vi "write_all_conditions_to_ini.vi"() -> ()   [LabVIEW 2019]
uses:
  <vilib>/Utility/config.llb/NI_LVConfig.lvlib
panel:
  in  "Conditions cluster":T1
  in  "configuration file path":path
  in  "Error in":errorcluster
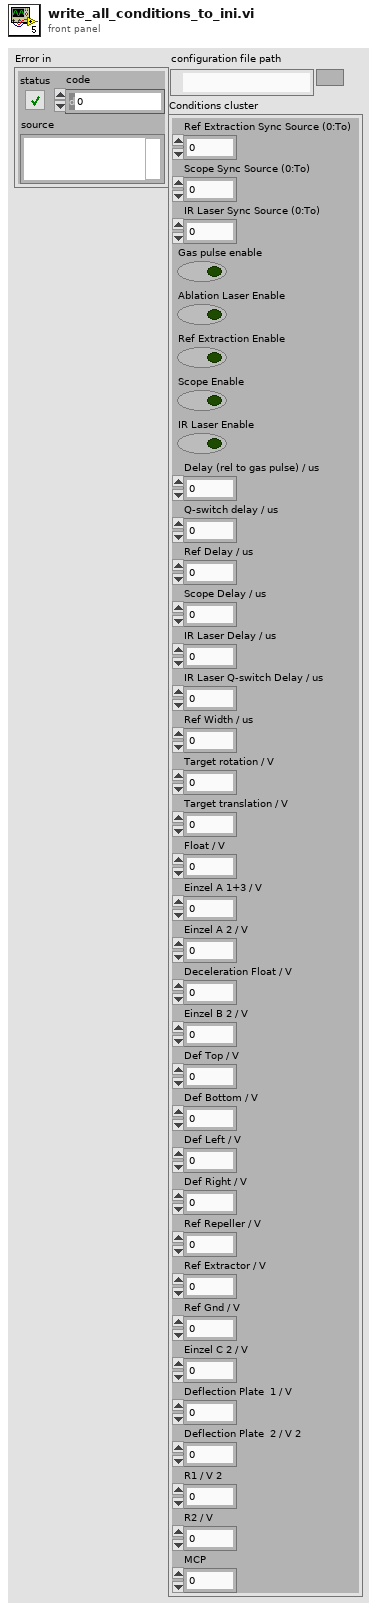
[diagram p1: front panel]
types:
  T1 = cluster{"Ref Extraction Sync Source (0:To)":i32, "Scope Sync Source (0:To)":i32, "IR Laser Sync Source (0:To)":i32, "Gas pulse enable":bool, "Ablation Laser Enable":bool, "Ref Extraction Enable":bool, "Scope Enable":bool, "IR Laser Enable":bool, "Delay (rel to gas pulse) / us":dbl, "Q-switch delay / us":dbl, "Ref Delay / us":dbl, "Scope Delay / us":dbl, "IR Laser Delay / us":dbl, "IR Laser Q-switch Delay / us":dbl, "Ref Width / us":dbl, "Target rotation / V":dbl, "Target translation / V":dbl, "Float / V":dbl, "Einzel A 1+3 / V":dbl, "Einzel A 2 / V":dbl, "Deceleration Float / V":dbl, "Einzel B 2 / V":dbl, "Def Top / V":dbl, "Def Bottom / V":dbl, "Def Left / V":dbl, "Def Right / V":dbl, "Ref Repeller / V":dbl, "Ref Extractor / V ":dbl, "Ref Gnd / V ":dbl, "Einzel C 2 / V":dbl, "Deflection Plate  1 / V":dbl, "Deflection Plate  2 / V 2":dbl, "R1 / V 2":dbl, "R2 / V":dbl, "MCP":dbl}
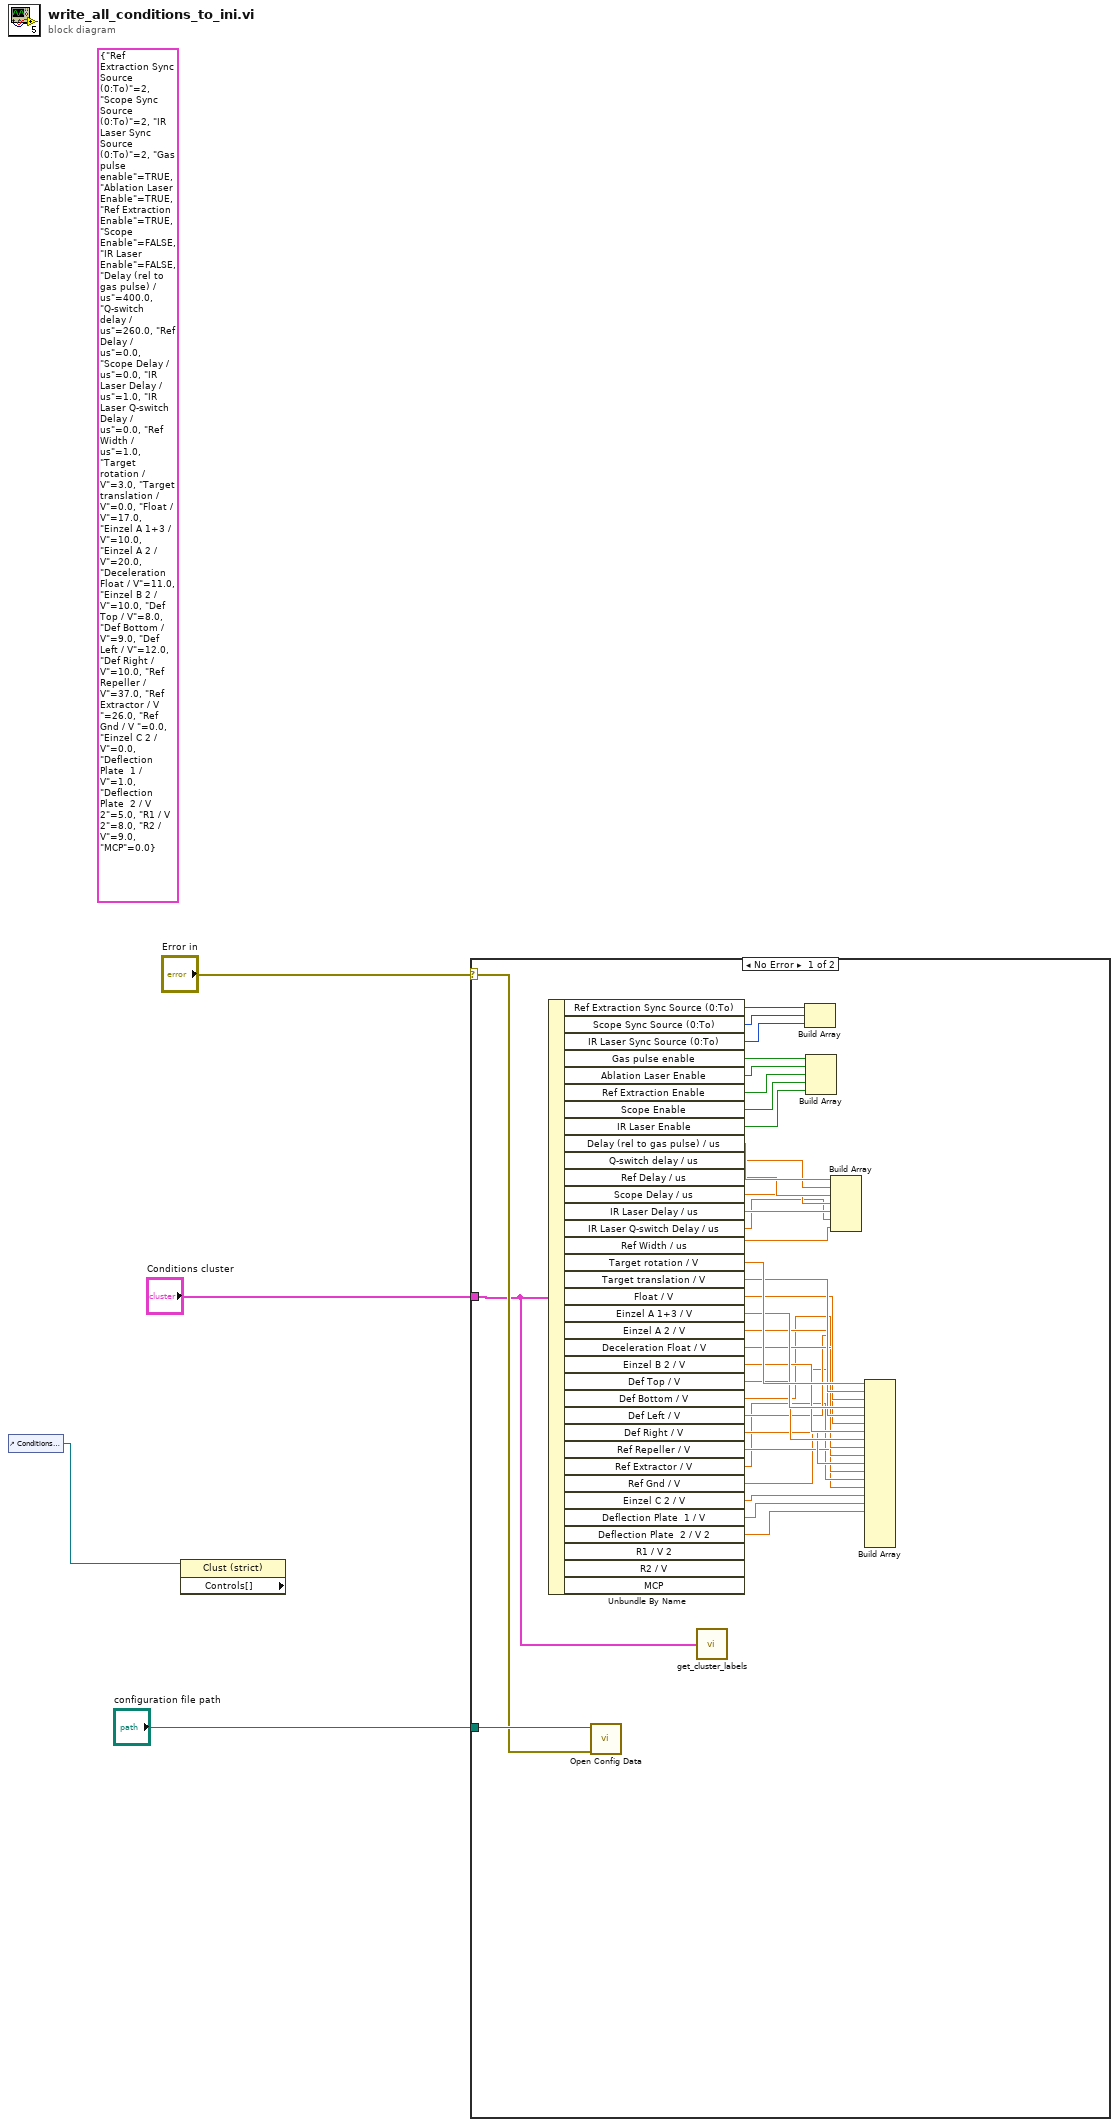
[diagram p0: block diagram]
diagram:
  (unwired) T1 {"Ref Extraction Sync Source (0:To)"=2, "Scope Sync Source (0:To)"=2, "IR Laser Sync Source (0:To)"=2, "Gas pulse enable"=TRUE, "Ablation Laser Enable"=TRUE, "Ref Extraction Enable"=TRUE, "Scope Enable"=FALSE, "IR Laser Enable"=FALSE, "Delay (rel to gas pulse) / us"=400.0, "Q-switch delay / us"=260.0, "Ref Delay / us"=0.0, "Scope Delay / us"=0.0, "IR Laser Delay / us"=1.0, "IR Laser Q-switch Delay / us"=0.0, "Ref Width / us"=1.0, "Target rotation / V"=3.0, "Target translation / V"=0.0, "Float / V"=17.0, "Einzel A 1+3 / V"=10.0, "Einzel A 2 / V"=20.0, "Deceleration Float / V"=11.0, "Einzel B 2 / V"=10.0, "Def Top / V"=8.0, "Def Bottom / V"=9.0, "Def Left / V"=12.0, "Def Right / V"=10.0, "Ref Repeller / V"=37.0, "Ref Extractor / V "=26.0, "Ref Gnd / V "=0.0, "Einzel C 2 / V"=0.0, "Deflection Plate  1 / V"=1.0, "Deflection Plate  2 / V 2"=5.0, "R1 / V 2"=8.0, "R2 / V"=9.0, "MCP"=0.0} ("input cluster")
  n1 = control-ref of="Conditions cluster"() -> (w1:refnum<vi>)
  n2 = property class="Clust (strict)" props=["Controls[]"](reference=w1) -> ()  [unwired: 1 in, 3 out]
  n3 = case shown="No Error" "Error in" {
    selector: "Error in" -> [w38 _]
    tunnel: "configuration file path" -> [w39 _]
    tunnel: "Conditions cluster" -> [w37 _]
    frame No Error {
      n4 = Unbundle By Name(w37) -> ("Ref Extraction Sync Source (0:To)"=w36:i32, "Scope Sync Source (0:To)"=w35:i32, "IR Laser Sync Source (0:To)"=w34:i32, "Gas pulse enable"=w33:bool, "Ablation Laser Enable"=w32:bool, "Ref Extraction Enable"=w31:bool, "Scope Enable"=w30:bool, "IR Laser Enable"=w29:bool, "Delay (rel to gas pulse) / us"=w28:dbl, "Q-switch delay / us"=w27:dbl, "Ref Delay / us"=w26:dbl, "Scope Delay / us"=w25:dbl, "IR Laser Delay / us"=w24:dbl, "IR Laser Q-switch Delay / us"=w23:dbl, "Ref Width / us"=w22:dbl, "Target rotation / V"=w21:dbl, "Target translation / V"=w20:dbl, "Float / V"=w19:dbl, "Einzel A 1+3 / V"=w18:dbl, "Einzel A 2 / V"=w17:dbl, "Deceleration Float / V"=w16:dbl, "Einzel B 2 / V"=w15:dbl, "Def Top / V"=w14:dbl, "Def Bottom / V"=w13:dbl, "Def Left / V"=w12:dbl, "Def Right / V"=w11:dbl, "Ref Repeller / V"=w10:dbl, "Ref Extractor / V"=w9:dbl, "Ref Gnd / V"=w8:dbl, "Einzel C 2 / V"=w7:dbl, "Deflection Plate  1 / V"=w6:dbl, "Deflection Plate  2 / V 2"=w5:dbl)  [unwired: 3 out]
      n5 = call <vilib>:"Open Config Data.vi"("error in (no error)"=w38, "configuration file path"=w39) -> ()  [unwired: 7 in, 3 out]
      n6 = call "get_cluster_labels.vi"("Conditions cluster"=w37) -> ()  [unwired: 1 out]
      n7 = Build Array(w36, w35, w34) -> ()  [unwired: 1 out]
      n8 = Build Array(w33, w32, w31, w30, w29) -> ()  [unwired: 1 out]
      n9 = Build Array(w28, w27, w26, w25, w24, w23, w22) -> ()  [unwired: 1 out]
      n10 = Build Array(w21, w20, w19, w18, w17, w16, w15, w14, w13, w12, w11, w10, w9, w8, w7, w6, w5) -> ()  [unwired: 4 in, 1 out]
    }
    frame Error {
    }
  }
